vi "End_of_run_messages.vi"(0 "Message":string, 2 "Subject":string, 3 "Attachments":string[](array[string])) -> ()   [LabVIEW 2010]
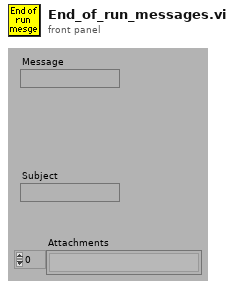
[diagram p1: front panel]
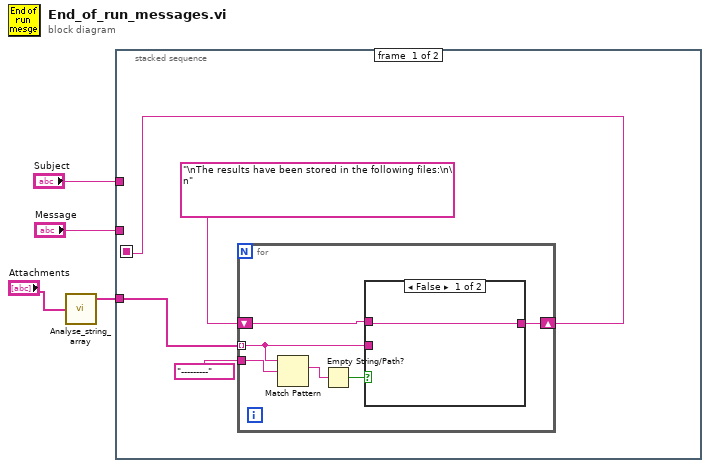
[diagram p0: block diagram]
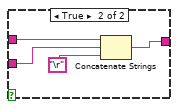
[diagram p2: hidden frame]
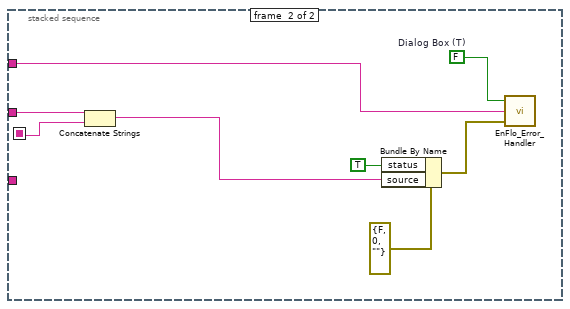
[diagram p3: hidden frame]
diagram:
  n1 = call "Analyse_string_array.vi"("String array"="Attachments") -> ("Unique strings"=w1:string[])  [unwired: 2 out]
  n2 = stacked-sequence {
    seq-local: [w6 _] -> [_ w26]
    tunnel: "Message" -> [_ w27]
    tunnel: "Subject" -> [_ w21]
    tunnel: w1 -> [w8 _]
    frame #0 {
      n3 = for {
        shift-right: [w13] -> w6
        shift-left: "\nThe results have been stored in the following files:\n\n" -> [w14]
        tunnel: w8 -> [w11] mode=indexing
        tunnel: "---------" -> [w12]
        n4 = Match Pattern(string=w11, regular expression=w12) -> (match substring=w10:string)  [unwired: 4 out]
        n5 = Empty String/Path?(string/path=w10) -> (empty?=w9:bool)
        n6 = case shown="False" w9 {
          tunnel: w14 -> [w15 w19]
          tunnel: [w15 w18] -> w13
          tunnel: w11 -> [_ w17]
          frame False {
          }
          frame True {
            n7 = Concatenate Strings(w19, w17, "\r") -> (w18:string)
          }
        }
      }
    }
    frame #1 {
      w20 = FALSE  # Dialog Box (T)
      n8 = Concatenate Strings(w27, w26) -> (w23:string)
      n9 = Bundle By Name(cluster=errorcluster {"status"=FALSE, "code"=0, "source"=""} ("error in (no error)"), "status"=TRUE ("Bundle Element"), "source"=w23) -> (w22:errorcluster)
      n10 = call "EnFlo_Error_Handler.vi"("error in (no error)"=w22, "Error Type"=w21, "Dialog Box (T)"=w20) -> ()  [unwired: 3 out]
    }
  }
